vi "Get axis info.vi"(8 "error in":errorcluster, 9 "axis":u8, 10 "deviceHandle":u64, 11 "path in":path) -> (0 "error out":errorcluster, 1 "axis out":u8, 2 "deviceHandle out":u64, 3 "Axis info":T1 {"Index" items=["1", "2", "3"]; "ActuatorType" items=["Linear", "Rotator", "Goniometer"]})   [LabVIEW 2022 SP3, in "SampleRotator.lvlib"]
doc: "Queries axis (actuator) status, actual position, and current settings of amplitude, frequency.\n\ninputs: \npath to DLL; handle; axis; error cluster\n\noutputs:\nhandle; axis; axis status; error cluster"
uses:
  SampleRotator.lvlib
  ctl/Axis status.ctl
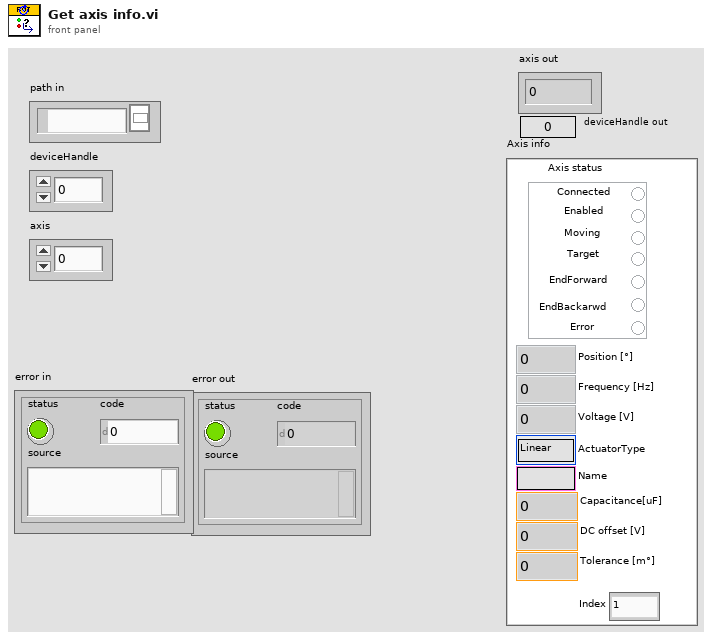
[diagram p1: front panel]
types:
  T1 = typedef "SampleRotator.lvlib/Axis status.ctl" = cluster{"Axis status":cluster{"Connected":bool, "Enabled":bool, "Moving":bool, "Target":bool, "EndForward":bool, "EndBackarwd":bool, "Error":bool}, "Position [°]":dbl, "Frequency [Hz]":dbl, "Voltage [V]":dbl, "Capacitance[uF]":dbl, "Name":string, "ActuatorType":u16, "DC offset [V]":dbl, "Tolerance [m°]":dbl, "Index":u8}
  T2 = cluster{"connected":bool, "enabled":bool, "moving":bool, "target":bool, "EotFwd":bool, "EotBwd":bool, "error":bool}
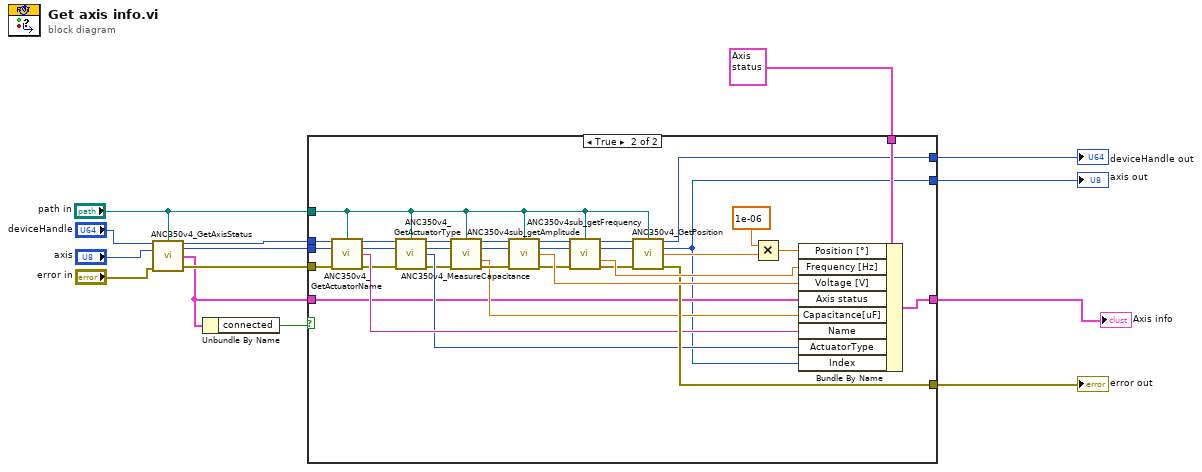
[diagram p0: block diagram]
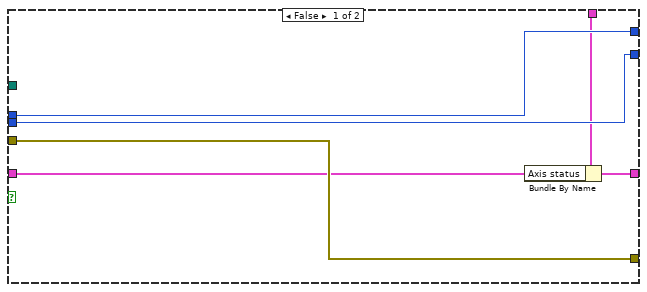
[diagram p2: hidden frame]
diagram:
  n1 = call <instrlib>:"ANC350v4_GetAxisStatus.vi"("deviceHandle"="deviceHandle", "Path to *.DLL"="path in", "axis"="axis", "error in"="error in") -> ("deviceHandle"=w4:u64, "axis"=w3:u8, "Axis status"=w2:T2, "error ANC350v4_getAxisStatus"=w6:errorcluster)  [unwired: 7 in, 1 out]
  n2 = Unbundle By Name(w2) -> ("connected"=w1:bool)
  n3 = case shown="True" w1 {
    tunnel: [w16 w53] -> w14
    tunnel: T1 {"Axis status"={"Connected"=FALSE, "Enabled"=FALSE, "Moving"=FALSE, "Target"=FALSE, "EndForward"=FALSE, "EndBackarwd"=FALSE, "Error"=FALSE}, "Position [°]"=0.0, "Frequency [Hz]"=0.0, "Voltage [V]"=0.0, "Capacitance[uF]"=0.0, "Name"="", "ActuatorType"=0, "DC offset [V]"=0.0, "Tolerance [m°]"=0.0, "Index"=0} ("Axis info") -> [w18 w52]
    tunnel: [w20 w46] -> w12
    tunnel: [w17 w39] -> w11
    tunnel: [w19 w21] -> w10
    tunnel: "path in" -> [_ w26]
    tunnel: w6 -> [w17 w25]
    tunnel: w4 -> [w20 w24]
    tunnel: w3 -> [w19 w23]
    tunnel: w2 -> [w15 w22]
    frame False {
      n4 = Bundle By Name(cluster=w18, "Axis status"=w15) -> (w16:T1)
    }
    frame True {
      n5 = call <instrlib>:"ANC350v4_GetActuatorName.vi"("deviceHandle"=w24, "Path to *.DLL"=w26, "axis"=w23, "error in"=w25) -> ("deviceHandle"=w38:u64, "axis"=w37:u32, "ActuatorName"=w36:string, "error ANC350v4_getActuatorName"=w34:errorcluster)  [unwired: 8 in]
      n6 = call <instrlib>:"ANC350v4_GetActuatorType.vi"("deviceHandle"=w38, "Path to *.DLL"=w26, "axis"=w37, "error in"=w34) -> ("deviceHandle"=w33:u64, "axis"=w32:u32, "ActuatorType"=w35:u16, "error ANC350v4_getActuatorType"=w31:errorcluster)  [unwired: 8 in]
      n7 = call <instrlib>:"ANC350v4_MeasureCapacitance.vi"("deviceHandle"=w33, "Path to *.DLL"=w26, "axis"=w32, "error in"=w31) -> ("deviceHandle"=w29:u64, "axis"=w28:u8, "Capacitance"=w27:dbl, "error ANC350v4_frequency"=w30:errorcluster)  [unwired: 8 in]
      n8 = call <instrlib>:"ANC350v4sub_getAmplitude.vi"("deviceHandle"=w29, "Path to *.DLL"=w26, "axis"=w28, "error in"=w30) -> ("deviceHandle"=w47:u64, "axis"=w43:u8, "amplitude out"=w50:dbl, "error ANC350v4_Amplitude"=w45:errorcluster)  [unwired: 8 in]
      n9 = call <instrlib>:"ANC350v4sub_getFrequency.vi"("deviceHandle"=w47, "Path to *.DLL"=w26, "axis"=w43, "error in"=w45) -> ("deviceHandle"=w48:u64, "axis"=w42:u8, "Frequency [Hz] out"=w49:dbl, "error ANC350v4_frequency"=w44:errorcluster)  [unwired: 8 in]
      n10 = call <instrlib>:"ANC350v4_GetPosition.vi"("deviceHandle"=w48, "Path to *.DLL"=w26, "axis"=w42, "error in"=w44) -> ("deviceHandle"=w46:u64, "axis"=w21:u8, "Position [µm | m°]"=w51:dbl, "error ANC350v4_getPosition"=w39:errorcluster)  [unwired: 8 in]
      n11 = Multiply(x=1e-06, y=w51) -> (x*y=w41:dbl)
      n12 = Bundle By Name(cluster=w52, "Position [°]"=w41, "Frequency [Hz]"=w49, "Voltage [V]"=w50, "Axis status"=w22, "Capacitance[uF]"=w27, "Name"=w36, "ActuatorType"=w35, "Index"=w21) -> (w53:T1)
    }
  }
  "Axis info" <- w14
  "error out" <- w11
  "deviceHandle out" <- w12
  "axis out" <- w10
